vi "TInScan.VI"(0 "LowChan":u32, 1 "HighChan":u32, 2 "Scale(Celsius)":u32(ring) items=["CELSIUS", "FAHRENHEIT", "KELVIN"], 3 "Options (FILTER)":bool=TRUE, 4 "BoardNum (0)":u32 max=8) -> (5 "DataValues":sgl[](array[numeric]) format="%.2f", 6 "ErrCode":i32)   [LabVIEW 2019, in "DAQ_Engine.lvclass"]
doc: "Developed by Kevin Thompson\nkevin@thompsonengineering.net\n\nCopyright 2020\nThompson Engineering, LLC\nReads a range of channels from an analog input board, linearizes the measurements according to temperature sensor type, and returns the temperatures to array."
uses:
  DAQ_Engine.lvclass
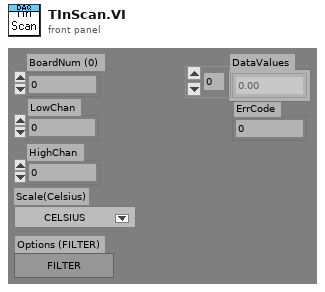
[diagram p1: front panel]
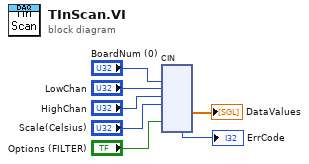
[diagram p0: block diagram]
diagram:
  n1 = cin("BoardNum (0)", "LowChan", "HighChan", "Scale(Celsius)", "Options (FILTER)") -> (→"DataValues":sgl[], →"ErrCode":i32)  [unwired: 7 in]
